vi "Set NATS Connection.vi"(8 "error in":errorcluster {"code" format="Error %.0f"}, 10 "NATS Connection":T1={"connection ID"=refnum, "server INFO"="", "timeout ms"=5000, "verbose?"=FALSE, "server headers?"=FALSE, "client headers?"=FALSE}, 11 "NATS Client.lvlib:NATS Client.lvclass":refnum<class "NATS Client.lvclass">) -> (0 "error out":errorcluster, 3 "NATS Client out":refnum<class "NATS Client.lvclass">)   [LabVIEW 2024, in "NATS Client.lvlib" / "NATS Client.lvclass"]
uses:
  NATS Client.lvclass
  NATS Client.lvclass/NATS Client.ctl
  <vilib>/NATS/NATS Core/Controls/nats connection.ctl
  <vilib>/NATS/NATS Core/NATS Core.lvlib
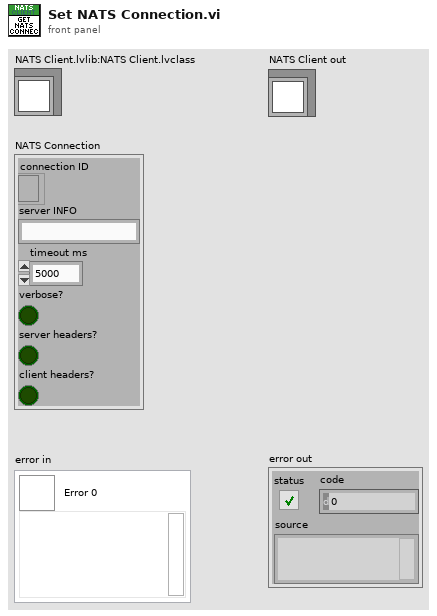
[diagram p1: front panel]
types:
  T1 = typedef "NATS Core.lvlib/nats connection.ctl" = cluster{"connection ID":refnum<k5>, "server INFO":string, "timeout ms":i32, "verbose?":bool, "server headers?":bool, "client headers?":bool}
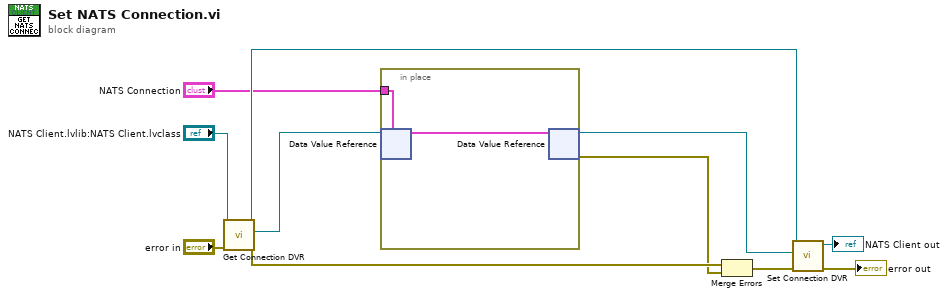
[diagram p0: block diagram]
diagram:
  n1 = call "Get Connection DVR.vi"("error in"="error in", "NATS Client in"="NATS Client.lvlib:NATS Client.lvclass") -> ("error out"=w9:errorcluster, "NATS Connection"=w10:refnum<data-value>, "NATS Client out"=w4:refnum<class "NATS Client.lvclass">)  [unwired: 7 in]
  n2 = in-place {
    in-place-border: "NATS Connection" -> [w12]
    n3 = in-place-dvr #1(w10) -> ()  [unwired: 2 out]
    n4 = in-place-dvr #1(w12) -> (w2:refnum<data-value>, w7:errorcluster)
  }
  n5 = Merge Errors(w9, w7) -> (w6:errorcluster)
  n6 = call "Set Connection DVR.vi"("error in"=w6, "NATS Connection"=w2, "NATS Client in"=w4) -> ("error out"=→"error out":errorcluster, "NATS Client out"=→"NATS Client out":refnum<class "NATS Client.lvclass">)  [unwired: 7 in]
